vi "Keithley6487 Read.vi"(7 "Enable Zero Correction":bool=TRUE, 8 "error in":errorcluster, 9 "Voltage (V)":dbl, 10 "Sample per measurement":u32=1 max=2500, 11 "VISA in":refnum<visa-resource-name>="COM3") -> (0 "error out":errorcluster, 1 "Zero Offset":string, 2 "Current (A)":dbl, 3 "VISA out":refnum<visa-resource-name>)   [LabVIEW 2018]
uses:
  <vilib>/Analysis/NI_AALBase.lvlib
  <vilib>/Analysis/baseanly.llb/Mean (DBL).vi
panel:
  in  "Zero Correction Procedure":string=":TRIG:COUN 1;:SYST:ZCH 1;:CURR:RANG 2E-9;:INIT;:SYST:ZCOR 0;:SYST:ZCOR:ACQ;:SYST:ZCH 0;:SYST:ZCOR 1;:CURR:RANG 2E-2;:FETC?"
  in  "Error procedure":string
  out "read buffer":string
  in  "Bytes to Read":i32=40000
  # "Error out reports Serial I/O errors.\n\nKeithley Error reports error messages returned by the Keithley 6485 picoAmmeter.  Currently, only overvoltage and invalid data errors are supported by this VI."
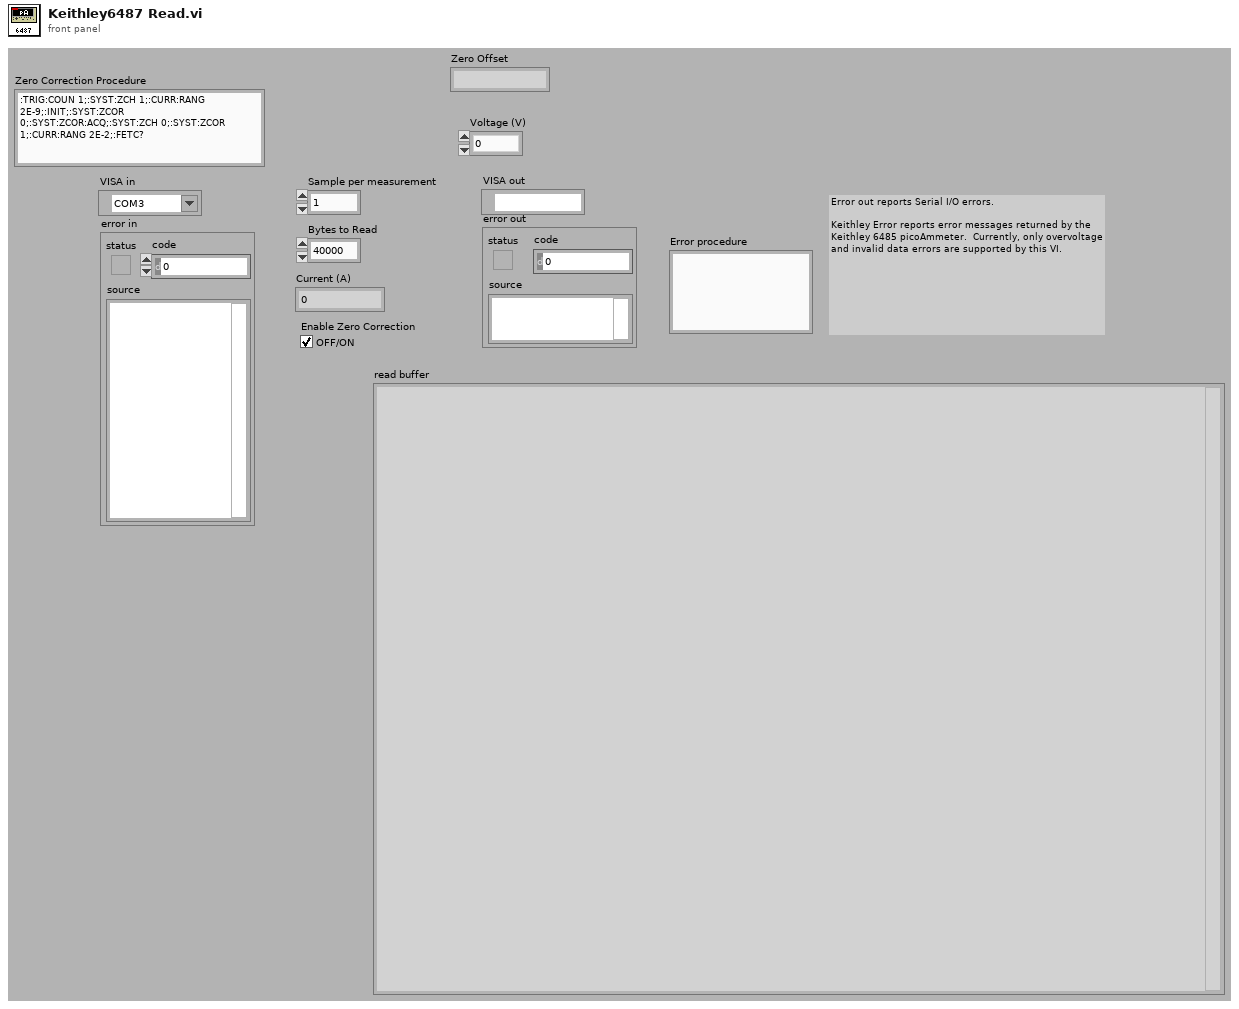
[diagram p1: front panel]
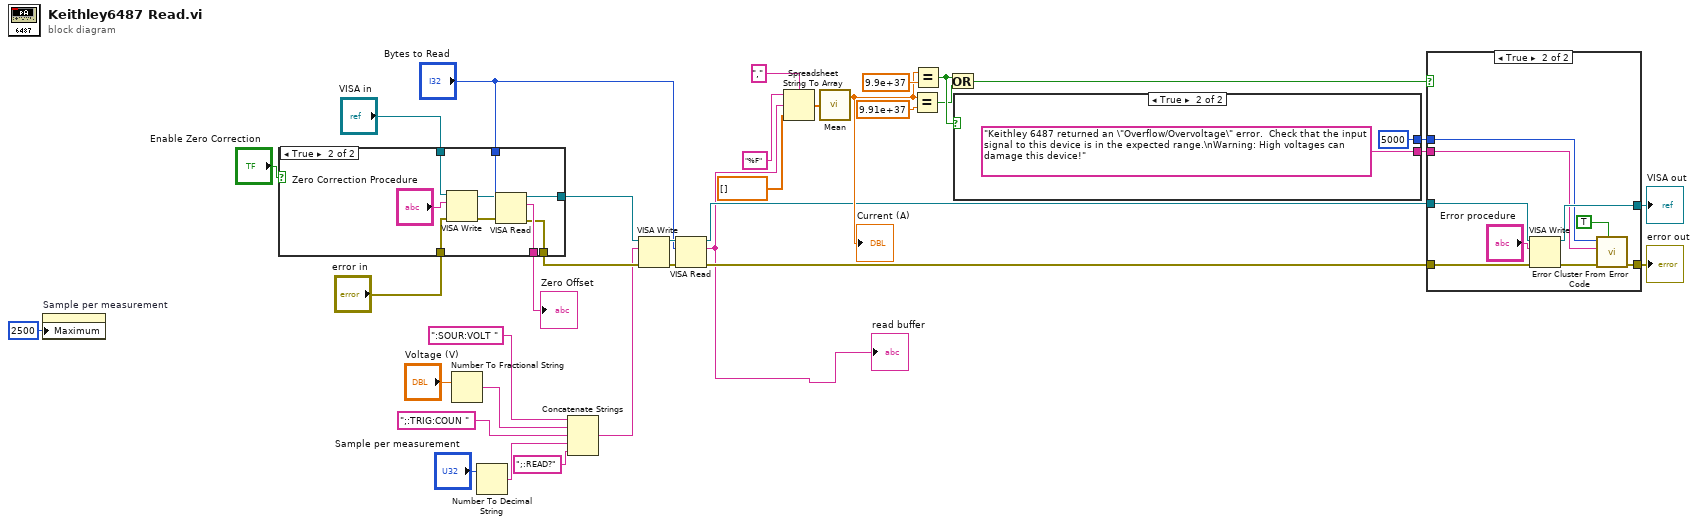
[diagram p0: block diagram]
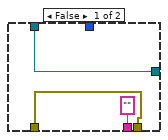
[diagram p2: hidden frame]
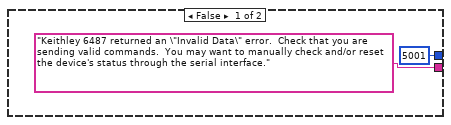
[diagram p3: hidden frame]
diagram:
  n1 = property on="Sample per measurement" class="DigNum (strict)"("Maximum"=u32 2500 ("Data Entry Limits:Maximum")) -> ()  [unwired: 2 in, 2 out]
  n2 = case shown="True" "Enable Zero Correction" {
    tunnel: "VISA in" -> [w37 w46]
    tunnel: "error in" -> [w36 w45]
    tunnel: "Bytes to Read" -> [_ w44]
    tunnel: ["" ("read buffer") w41] -> w4
    tunnel: [w37 w40] -> w3
    tunnel: [w36 w39] -> w2
    frame False {
    }
    frame True {
      n3 = VISA Write(VISA resource name=w46, write buffer="Zero Correction Procedure", error in (no error)=w45) -> (VISA resource name out=w43:refnum<visa-resource-name>, error out=w42:errorcluster)  [unwired: 1 out]
      n4 = VISA Read(VISA resource name=w43, byte count=w44, error in (no error)=w42) -> (VISA resource name out=w40:refnum<visa-resource-name>, read buffer=w41:string, error out=w39:errorcluster)  [unwired: 1 out]
    }
  }
  "Zero Offset" <- w4
  n5 = Number To Fractional String(number="Voltage (V)") -> (F-format string=w9:string)  [unwired: 3 in]
  n6 = Number To Decimal String(number="Sample per measurement") -> (decimal integer string=w32:string)  [unwired: 1 in]
  n7 = Concatenate Strings(":SOUR:VOLT ", w9, ";:TRIG:COUN ", w32, ";:READ?") -> (w1:string)
  n8 = VISA Write(VISA resource name=w3, write buffer=w1, error in (no error)=w2) -> (VISA resource name out=w34:refnum<visa-resource-name>, error out=w35:errorcluster)  [unwired: 1 out]
  n9 = VISA Read(VISA resource name=w34, byte count="Bytes to Read", error in (no error)=w35) -> (VISA resource name out=w21:refnum<visa-resource-name>, read buffer=w8:string, error out=w20:errorcluster)  [unwired: 1 out]
  "read buffer" <- w8
  n10 = Spreadsheet String To Array(delimiter (Tab)=",", format string="%F", spreadsheet string=w8, array type (2D Dbl)=dbl[] [] ("Array")) -> (array=w27:dbl[])
  n11 = call-poly <vilib>:"Mean.vi"("X"=w27) -> ("mean"=w22:dbl)  [unwired: 1 out]
  "Current (A)" <- w22
  n12 = Equal?(x=w22, y=9.91e+37) -> (x = y?=w16:bool)
  n13 = Equal?(x=w22, y=9.9e+37) -> (x = y?=w17:bool)
  n14 = Or(x=w17, y=w16) -> (x .or. y?=w18:bool)
  n15 = case shown="True" w17 {
    tunnel: ["Keithley 6487 returned an \"Invalid Data\" error.  Check that you are sending valid commands.  You may want to manually check and/or reset the device's status through the serial interface." "Keithley 6487 returned an \"Overflow/Overvoltage\" error.  Check that the input signal to this device is in the expected range.\nWarning: High voltages can damage this device!"] -> w13
    tunnel: [5001 ("error code (0)") 5000 ("error code (0)")] -> w12
    frame False {
    }
    frame True {
    }
  }
  n16 = case shown="True" w18 {
    tunnel: w21 -> [w53 w62]
    tunnel: w20 -> [w52 w61]
    tunnel: [w53 w60] -> w19
    tunnel: [w52 w57] -> w14
    tunnel: w13 -> [_ w56]
    tunnel: w12 -> [_ w54]
    frame False {
    }
    frame True {
      n17 = VISA Write(VISA resource name=w62, write buffer="Error procedure", error in (no error)=w61) -> (VISA resource name out=w60:refnum<visa-resource-name>, error out=w58:errorcluster)  [unwired: 1 out]
      n18 = call <vilib>:"Error Cluster From Error Code.vi"("show call chain? (False)"=TRUE, "error in (no error)"=w58, "error message (\"\")"=w56, "error code (0)"=w54) -> ("error out"=w57:errorcluster)  [unwired: 5 in]
    }
  }
  "VISA out" <- w19
  "error out" <- w14
